vi "zs_prologer.vi"(7 "node_goal":string="b505", 9 "y":dbl=300.0, 10 "x":dbl=520.0) -> (3 "goal_array":T1(array[cluster]))   [LabVIEW 2014, in "Dialogue.lvlib" / "Dialogue.lvclass"]
uses:
  Dialogue.lvclass
  <vilib>/regexp/Match Regular Expression.xnode
panel:
  out "坐标数组":dbl[][](array[numeric])
  out "添加的路径":path
  out "数组":string[][](array[string])
  out "结果字符串":string
  out "standard output":string caption="标准输出"
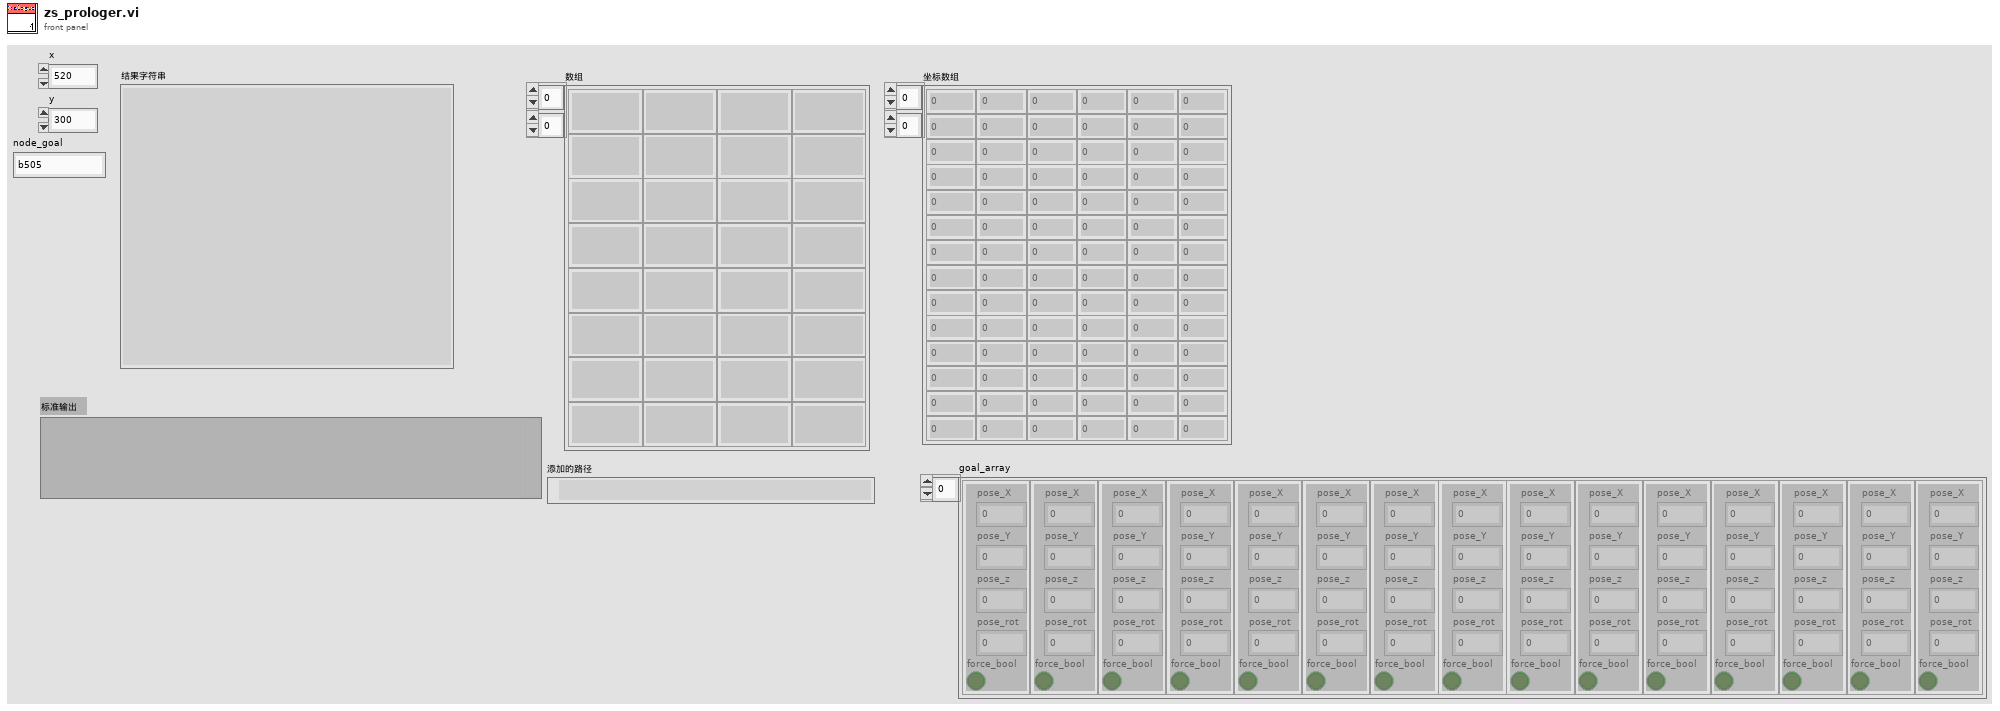
[diagram p1: front panel]
types:
  T1 = cluster{"pose_X":dbl, "pose_Y":dbl, "pose_z":dbl, "pose_rot":dbl, "force_bool":bool}[]
  T2 = cluster{"pose_X":dbl, "pose_Y":dbl, "pose_z":dbl, "pose_rot":dbl, "force_bool":bool}
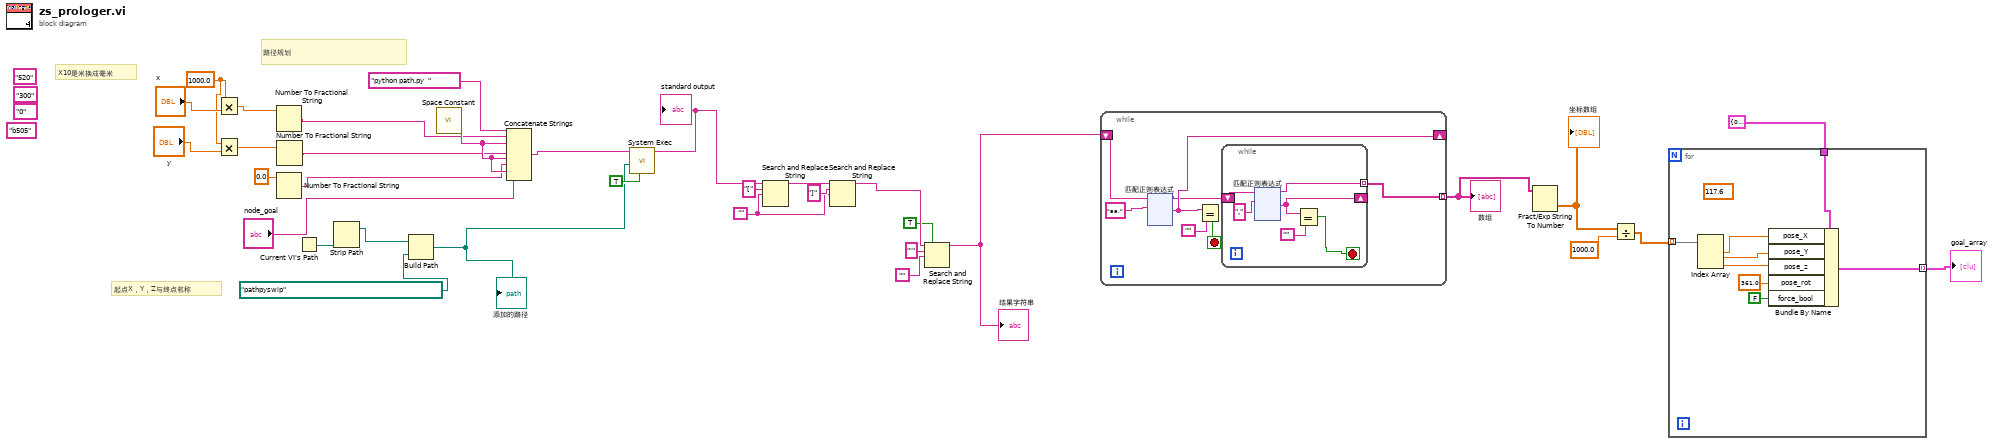
[diagram p0: block diagram]
diagram:
  w6 = 1000.0 ("x")
  (unwired) "b505" ("元素")
  (unwired) "0" ("元素")
  (unwired) "300" ("元素")
  (unwired) "520" ("元素")
  w27 = ""
  # "X10是米换成毫米"
  # "起点X，Y，Z与终点名称"
  # "路径规划"
  n1 = Multiply(x=w6, y="x") -> (x*y=w5:dbl)
  n2 = Multiply(x=w6, y="y") -> (x*y=w4:dbl)
  n3 = Number To Fractional String(number=w5) -> (F-format string=w16:string)  [unwired: 3 in]
  n4 = Number To Fractional String(number=0.0 ("数字")) -> (F-format string=w13:string)  [unwired: 3 in]
  n5 = Number To Fractional String(number=w4) -> (F-format string=w15:string)  [unwired: 3 in]
  n6 = Current VI's Path() -> (path=w21:path)
  n7 = Strip Path(path=w21) -> (stripped path=w19:path)  [unwired: 1 out]
  n8 = Build Path(base path=w19, name or relative path=path "pathpyswip") -> (appended path=w17:path)
  "添加的路径" <- w17
  n9 = call <vilib>:"Space Constant.vi"() -> ("String"=w33:string)
  n10 = Concatenate Strings("python path.py  " ("command line"), w16, w33, w15, w33, w13, w33, "node_goal") -> (w32:string)
  n11 = call <vilib>:"System Exec.vi"("run minimized? (F)"=TRUE, "working directory"=w17, "command line"=w32) -> ("standard output"=w31:string)  [unwired: 5 in, 3 out]
  "standard output" <- w31
  n12 = Search and Replace String(input string=w31, search string="[" ("搜索字符串"), replace string=w27) -> (result string=w29:string)  [unwired: 5 in, 3 out]
  n13 = Search and Replace String(input string=w29, search string="]" ("搜索字符串"), replace string=w27) -> (result string=w26:string)  [unwired: 5 in, 3 out]
  n14 = Search and Replace String(replace all?=TRUE ("替换全部？(F)"), input string=w26, search string="'" ("搜索字符串"), replace string="") -> (result string=w22:string)  [unwired: 4 in, 3 out]
  "结果字符串" <- w22
  n15 = while {
    tunnel: [w35] -> w11 mode=indexing
    shift-right: [w39] -> _
    shift-left: w22 -> [w40]
    stop <- w37 stop-if-true
    n16 = xnode "匹配正则表达式"("输入字符串"=w40, "正则表达式"="aa,") -> ("匹配之前"=w36:string, "匹配之后"=w39:string)  [unwired: 4 in, 3 out]
    n17 = Equal?(x=w39, y="") -> (x = y?=w37:bool)
    n18 = while {
      shift-right: [w43] -> _
      shift-left: w36 -> [w47]
      tunnel: [w45] -> w35 mode=indexing
      stop <- w42 stop-if-true
      n19 = xnode "匹配正则表达式"("输入字符串"=w47, "正则表达式"=",") -> ("匹配之前"=w45:string, "匹配之后"=w43:string)  [unwired: 4 in, 3 out]
      n20 = Equal?(x=w43, y="") -> (x = y?=w42:bool)
    }
  }
  "数组" <- w11
  n21 = Fract/Exp String To Number(string=w11) -> (number=w2:dbl[][])  [unwired: 3 in, 1 out]
  "坐标数组" <- w2
  n22 = Divide(x=w2, y=1000.0) -> (x/y=w3:dbl[][])
  n23 = for {
    tunnel: T2 {"pose_X"=0.0, "pose_Y"=0.0, "pose_z"=0.0, "pose_rot"=0.0, "force_bool"=FALSE} ("goal_with_force") -> [w280]
    tunnel: [w278] -> w9 mode=indexing
    tunnel: w3 -> [w277] mode=indexing
    (unwired) 117.6 ("x")
    n24 = Index Array(array=w277) -> (element #1=w283:dbl, element #2=w276:dbl, element #3=w282:dbl)  [unwired: 3 in]
    n25 = Bundle By Name(cluster=w280, "pose_X"=w283, "pose_Y"=w276, "pose_z"=w282, "pose_rot"=361.0, "force_bool"=FALSE) -> (w278:T2)
  }
  "goal_array" <- w9
